vi "Power Sequence CSV Validity Check.vi"(8 "error in":errorcluster, 9 "Enable Validity Check?":bool, 10 "Extracted CSV":string[][](array[string]), 11 "File Path":path) -> (0 "error out":errorcluster, 2 "Valid Execution Order":bool, 3 "All Instruments Available":bool, 5 "Instruments not found":string[](array[string]))   [LabVIEW 2023]
doc: "Validates instrument availability and execution order using extracted CSV data.\n\nIf File Path is specified, the VI reads the CSV data from the file. If File Path is empty, the VI uses the data provided through the Extracted CSV input.\n\nInputs:\n- File Path: Path to the extracted CSV file. If empty, Extracted CSV is used.\n- Extracted CSV (2D String): CSV data provided directly as a 2D string array.\n- error in: Standard error cluster input.\n\nOutputs:\n- Instruments not found (1D String): List of instruments that were not found during validation.\n- All Instruments Available (Boolean): TRUE if all required instruments are found; otherwise FALSE.\n- Valid Execution Order (Boolean): TRUE if the execution order is valid; otherwise FALSE.\n- error out: Standard error cluster output."
uses:
  <vilib>/Utility/file.llb/Read Delimited Spreadsheet (string).vi
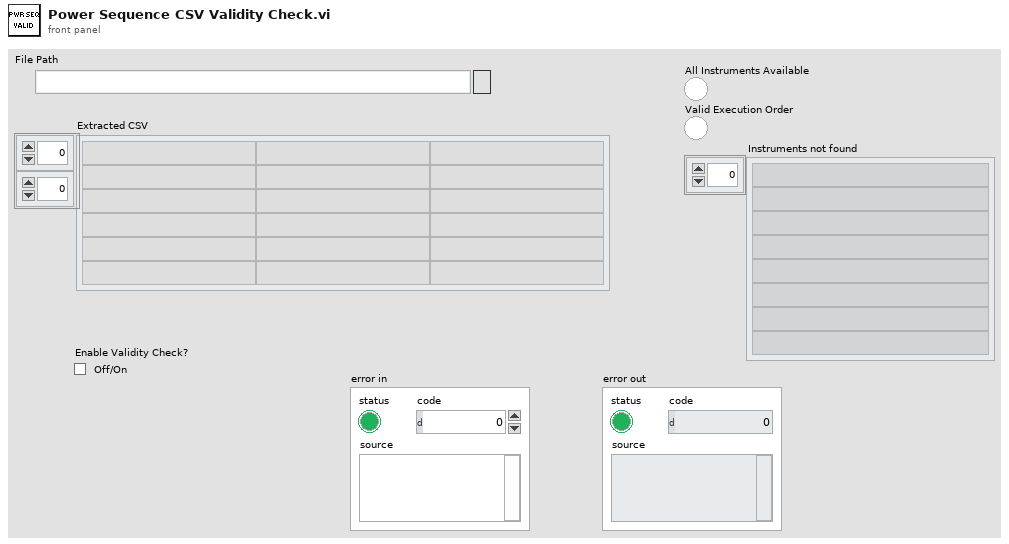
[diagram p1: front panel]
types:
  T1 = cluster{"Check":bool, "Execution Order Column Index":i32[]}
  T2 = cluster{"Section Name":string, "Instrument Column Index":i32, "Execution Order":cluster{"Check":bool, "Execution Order Column Index":i32[]}, "Extracted Configurations":string[][]}
  T3 = cluster{"Section Name":string, "Instrument Column Index":i32, "Execution Order":cluster{"Check":bool, "Execution Order Column Index":i32[]}, "Extracted Configurations":string[][]}[]
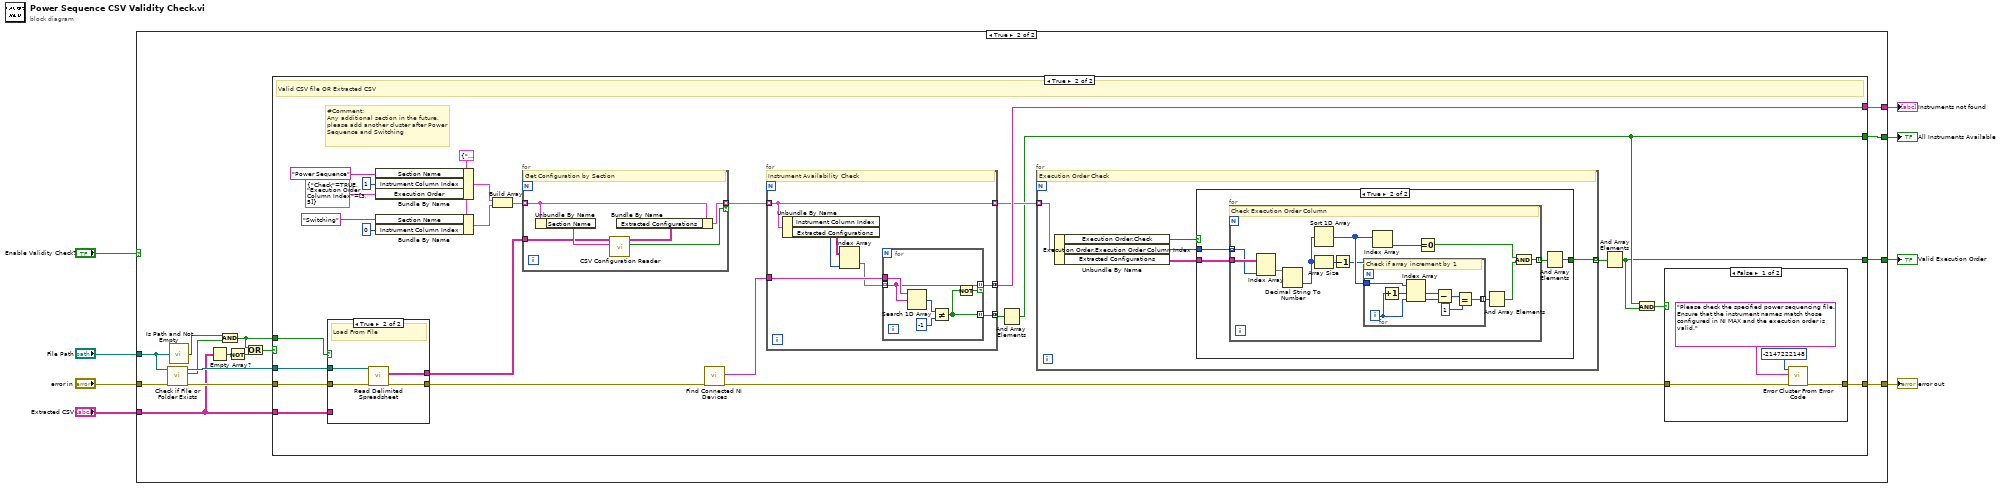
[diagram p0: block diagram]
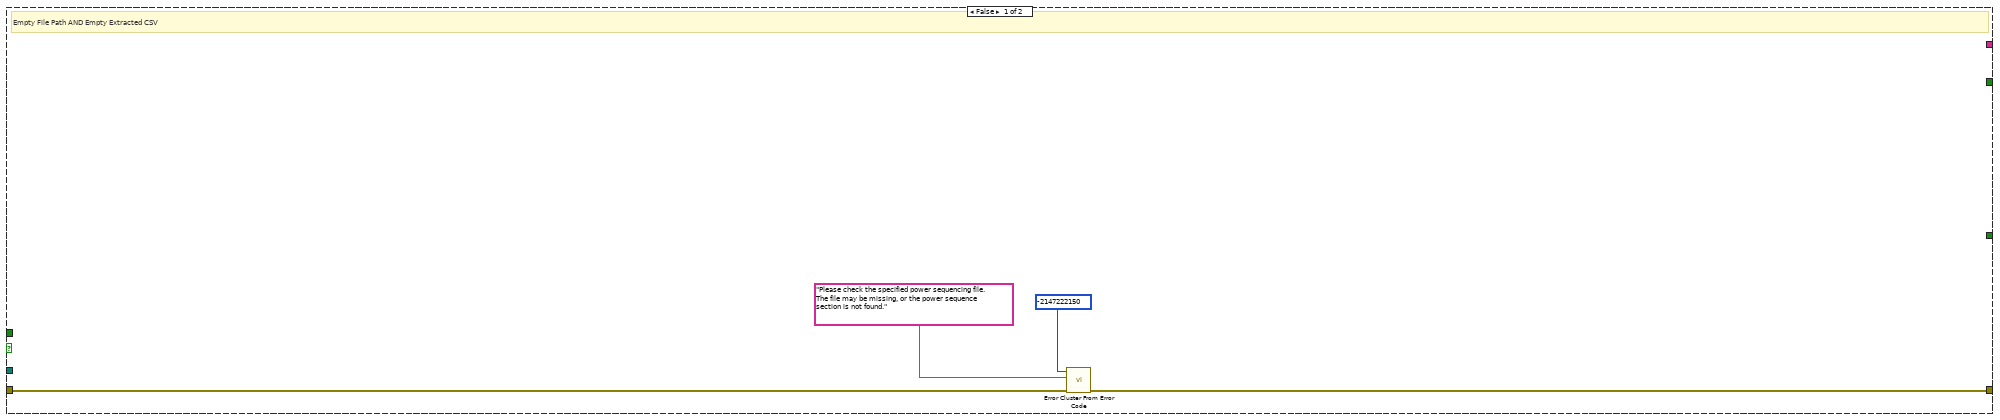
[diagram p3: hidden frame]
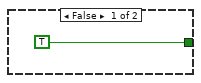
[diagram p5: hidden frame]
diagram:
  n1 = case shown="True" "Enable Validity Check?" {
    tunnel: "File Path" -> [_ w24]
    tunnel: [_ w22] -> w7
    tunnel: [_ w21] -> w6
    tunnel: [_ w20] -> w5
    tunnel: [w9 w19] -> w4
    tunnel: "error in" -> [w9 w18]
    tunnel: "Extracted CSV" -> [_ w12]
    frame False {
    }
    frame True {
      n2 = call <vilib>:"Check if File or Folder Exists.vi"("error in (no error)"=w18, "path"=w24) -> ("error out"=w23:errorcluster, "file or folder exists?"=w15:bool, "dup path"=w17:path)  [unwired: 7 in]
      n3 = call <vilib>:"Is Path and Not Empty.vi"("path"=w24) -> ("Is Path and Not Empty?"=w16:bool)  [unwired: 4 in]
      n4 = Empty Array?(array=w12) -> (empty?=w13:bool)
      n5 = And(x=w16, y=w15) -> (x .and. y?=w10:bool)
      n6 = Not(x=w13) -> (.not. x?=w11:bool)
      n7 = Or(x=w10, y=w11) -> (x .or. y?=w14:bool)
      n8 = case shown="True" w14 {
        tunnel: w17 -> [_ w54]
        tunnel: w23 -> [w26 w48]
        tunnel: [_ w46] -> w22
        tunnel: [_ w37] -> w21
        tunnel: [_ w36] -> w20
        tunnel: [w25 w34] -> w19
        tunnel: w12 -> [_ w38]
        tunnel: w10 -> [_ w32]
        frame False {
          # "Empty File Path AND Empty Extracted CSV"
          n9 = call <vilib>:"Error Cluster From Error Code.vi"("error in (no error)"=w26, "error message (\"\")"="Please check the specified power sequencing file. The file may be missing, or the power sequence section is not found.", "error code (0)"=-2147222150) -> ("error out"=w25:errorcluster)  [unwired: 6 in]
        }
        frame True {
          w29 = T2 {"Section Name"="", "Instrument Column Index"=0, "Execution Order"={"Check"=FALSE, "Execution Order Column Index"=[]}, "Extracted Configurations"=[]}
          # "#Comment:\nAny additional section in the future, please add another cluster after Power Sequence and Switching"
          # "Valid CSV file OR Extracted CSV"
          n10 = case shown="True" w32 {
            tunnel: w54 -> [_ w60]
            tunnel: w48 -> [w56 w59]
            tunnel: [w55 w58] -> w31
            tunnel: [w56 w57] -> w39
            tunnel: w38 -> [w55 _]
            frame False {
              # "Load from Extracted CSV"
            }
            frame True {
              # "Load From File"
              n11 = call-poly <vilib>:"Read Delimited Spreadsheet.vi"("file path (dialog if empty)"=w60, "error in (no error)"=w59) -> ("all rows"=w58:string[][], "error out"=w57:errorcluster)  [unwired: 8 in, 4 out]
            }
          }
          n12 = Bundle By Name(cluster=w29, "Section Name"="Power Sequence", "Instrument Column Index"=1, "Execution Order"=T1 {"Check"=TRUE, "Execution Order Column Index"=[3, 5]}) -> (w49:T2)
          n13 = Bundle By Name(cluster=w29, "Section Name"="Switching", "Instrument Column Index"=0) -> (w30:T2)
          n14 = Build Array(w49, w30) -> (w45:T3)
          n15 = for {
            tunnel: w45 -> [w64] mode=indexing
            tunnel: w31 -> [w65]
            tunnel: [w62] -> w44 mode=indexing if=w61
            # "Get Configuration by Section"
            n16 = Unbundle By Name(w64) -> ("Section Name"=w66:string)
            n17 = call "CSV Configuration Reader.vi"("Section"=w66, "All CSV Configurations"=w65) -> ("Section Exists?"=w61:bool, "Extracted Configurations"=w63:string[][])  [unwired: 8 in]
            n18 = Bundle By Name(cluster=w64, "Extracted Configurations"=w63) -> (w62:T2)
          }
          n19 = call "Find Connected NI Devices.vi"("error in"=w39) -> ("error out"=w35:errorcluster, "Alias Name(s)"=w47:string[])  [unwired: 8 in, 1 out]
          n20 = for {
            tunnel: w44 -> [w67] mode=indexing
            tunnel: w47 -> [w72]
            tunnel: [w70] -> w46 mode=concatenating
            tunnel: [w68] -> w43 mode=concatenating
            tunnel: [w67] -> w41 mode=indexing
            # "Instrument Availability Check"
            n21 = Unbundle By Name(w67) -> ("Instrument Column Index"=w73:i32, "Extracted Configurations"=w69:string[][])
            n22 = Index Array(array=w69, index (col)=w73) -> (element=w71:string[])  [unwired: 1 in]
            n23 = for {
              tunnel: w72 -> [w79]
              tunnel: w71 -> [w78] mode=indexing
              tunnel: [w75] -> w68 mode=indexing
              tunnel: [w78] -> w70 mode=indexing if=w74
              n24 = Search 1D Array(1D array=w79, element=w78) -> (index of element=w77:i32)  [unwired: 1 in]
              n25 = Not Equal?(x=w77, y=-1) -> (x != y?=w75:bool)
              n26 = Not(x=w75) -> (.not. x?=w74:bool)
            }
          }
          n27 = And Array Elements(Boolean array=w43) -> (logical AND=w37:bool)
          n28 = for {
            tunnel: w41 -> [w84] mode=indexing
            tunnel: [w80] -> w40 mode=indexing
            # "Execution Order Check"
            n29 = Unbundle By Name(w84) -> ("Execution Order.Check"=w83:bool, "Execution Order.Execution Order Column Index"=w81:i32[], "Extracted Configurations"=w82:string[][])
            n30 = case shown="True" w83 {
              tunnel: w82 -> [_ w89]
              tunnel: w81 -> [_ w88]
              tunnel: [TRUE w86] -> w80
              frame False {
              }
              frame True {
                n31 = for {
                  tunnel: w89 -> [w101]
                  tunnel: w88 -> [w99] mode=indexing
                  tunnel: [w90] -> w87 mode=indexing
                  # "Check Execution Order Column"
                  n32 = Index Array(array=w101, index (col)=w99) -> (element=w100:string[])  [unwired: 1 in]
                  n33 = Decimal String To Number(string=w100) -> (number=w95:i32[])  [unwired: 2 in, 1 out]
                  n34 = Sort 1D Array(array=w95) -> (sorted array=w96:i32[])
                  n35 = Array Size(array=w95) -> (size(s)=w97:i32)
                  n36 = Decrement(x=w97) -> (x-1=w91:i32)
                  n37 = for {
                    N: w91 -> [_]
                    tunnel: w96 -> [w109]
                    tunnel: [w102] -> w93 mode=indexing
                    i -> [w103]
                    # "Check if array increment by 1"
                    n38 = Increment(x=w103) -> (x+1=w104:i32)
                    n39 = Index Array(array=w109, index #1=w104, index #2=w103) -> (element #1=w108:i32, element #2=w107:i32)
                    n40 = Subtract(x=w108, y=w107) -> (x-y=w106:i32)
                    n41 = Equal?(x=w106, y=1) -> (x = y?=w102:bool)
                  }
                  n42 = Index Array(array=w96) -> (element=w98:i32)  [unwired: 1 in]
                  n43 = Equal To 0?(x=w98) -> (x = 0?=w94:bool)
                  n44 = And Array Elements(Boolean array=w93) -> (logical AND=w92:bool)
                  n45 = Compound Arithmetic op=AND(w94, w92) -> (w90:bool)
                }
                n46 = And Array Elements(Boolean array=w87) -> (logical AND=w86:bool)
              }
            }
          }
          n47 = And Array Elements(Boolean array=w40) -> (logical AND=w36:bool)
          n48 = And(x=w37, y=w36) -> (x .and. y?=w33:bool)
          n49 = case shown="False" w33 {
            tunnel: w35 -> [w111 w114]
            tunnel: [w110 w114] -> w34
            frame False {
              n50 = call <vilib>:"Error Cluster From Error Code.vi"("error in (no error)"=w111, "error message (\"\")"="Please check the specified power sequencing file. Ensure that the instrument names match those configured in NI MAX and the execution order is valid.", "error code (0)"=-2147222148) -> ("error out"=w110:errorcluster)  [unwired: 6 in]
            }
            frame True {
            }
          }
        }
      }
    }
  }
  "Instruments not found" <- w7
  "All Instruments Available" <- w6
  "Valid Execution Order" <- w5
  "error out" <- w4
